vi "Configure Contact Check Limit Test.vi"(7 "Contact Check Test Failure I/O Output (0)":u32, 8 "error in (no error)":errorcluster, 10 "Enable Contact Check Limit Test  (T:Enable)":bool=TRUE, 11 "VISA resource name":refnum<visa-resource-name>) -> (0 "error out":errorcluster, 3 "VISA resource name out":refnum<visa-resource-name>)   [LabVIEW 2022 SP3, in "Keithley 24XX.lvlib"]
doc: "Configures the contact check limit test (limit test #4).\n\n<B>Note:</B> This VI is only valid if your instrument has the contact check option available. Otherwise you will receive a \"Missing Hardware\" error, even if you are attempting to disable the test."
uses:
  Keithley 24XX.lvlib
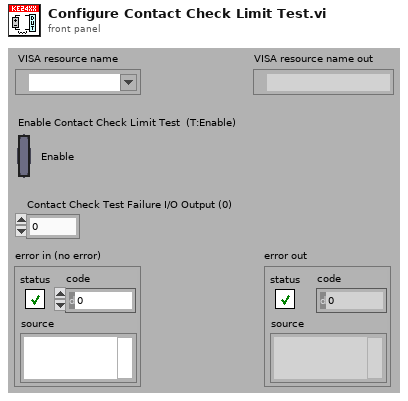
[diagram p1: front panel]
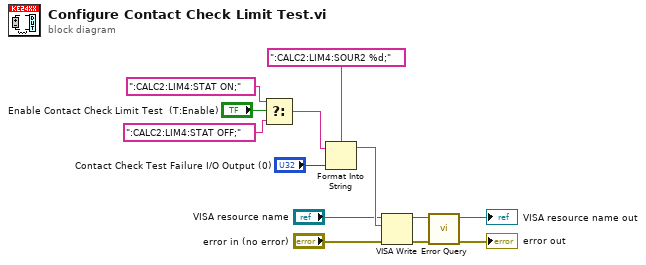
[diagram p0: block diagram]
diagram:
  n1 = Select(t=":CALC2:LIM4:STAT ON;", s="Enable Contact Check Limit Test  (T:Enable)", f=":CALC2:LIM4:STAT OFF;") -> (s? t:f=w3:string)
  n2 = Format Into String(format string=":CALC2:LIM4:SOUR2 %d;", initial string=w3, "Contact Check Test Failure I/O Output (0)") -> (resulting string=w9:string)  [unwired: 1 in, 1 out]
  n3 = VISA Write(VISA resource name="VISA resource name", write buffer=w9, error in (no error)="error in (no error)") -> (VISA resource name out=w11:refnum<visa-resource-name>, error out=w10:errorcluster)  [unwired: 1 out]
  n4 = call "Error Query.vi"("error in (no error)"=w10, "VISA resource name"=w11) -> ("error out"=→"error out":errorcluster, "VISA resource name out"=→"VISA resource name out":refnum<visa-resource-name>)  [unwired: 6 in, 2 out]
